vi "Position.vi"(0 "object in":refnum<class "5RobotsSkill.lvclass">, 2 "Robot":refnum<class "Robot.lvclass">, 4 "Game":refnum<class "Game.lvclass">, 5 "error in (no error)":errorcluster) -> (14 "object out":refnum<class "5RobotsSkill.lvclass">, 16 "Robot out":refnum<class "Robot.lvclass">, 19 "error out":errorcluster)   [LabVIEW 2024, in "5RobotsSkill.lvclass"]
uses:
  5RobotsSkill.lvclass
  Robot_class/Robot.lvclass
  Game_class/Game.lvclass
  Game_class/Game.lvclass/Game.ctl
  Robot_class/Robot.lvclass/Robot.ctl
  Robot_class/Read Zone.vi
  Robot_class/Write dest_orientation.vi
  Robot_class/Write dest_x.vi
  Robot_class/Write dest_y.vi
  Robot_class/Write kick_x.vi
  Robot_class/Write kick_z.vi
  Game_class/Read BallRef.vi
  Ball_class/Ball.lvclass
  Zone_class/Zone.lvclass
  Utilities_class/Utilities.lvclass
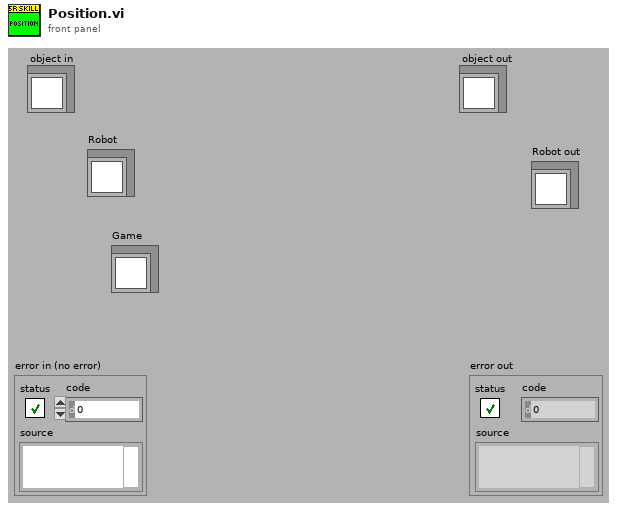
[diagram p1: front panel]
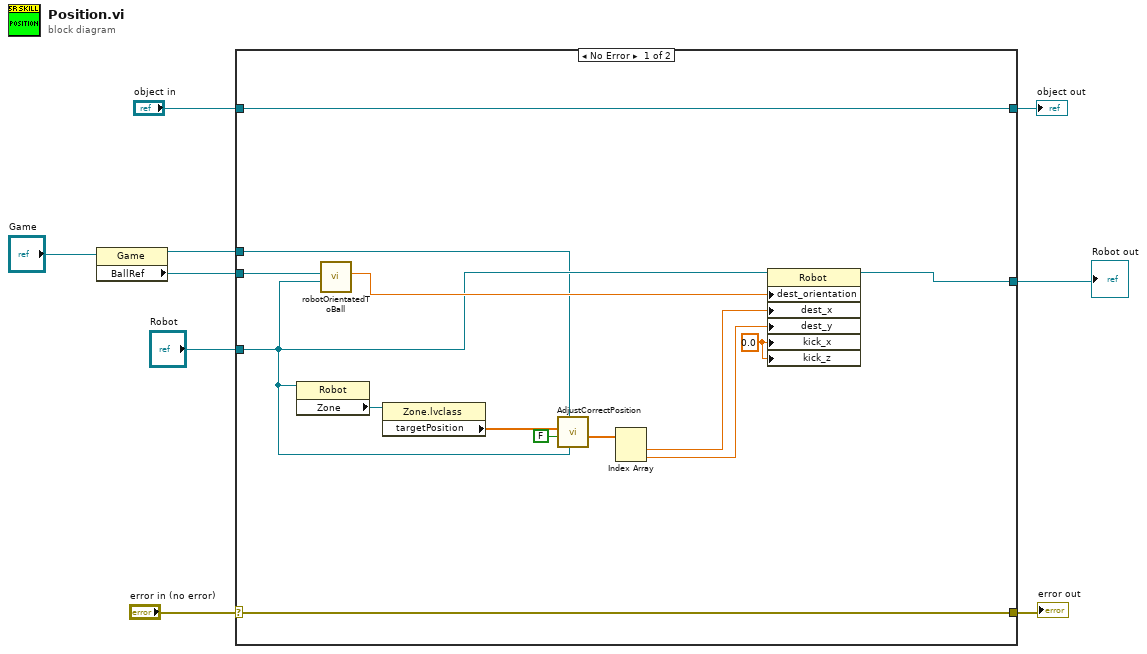
[diagram p0: block diagram]
diagram:
  n1 = property class="Game"(reference="Game") -> (reference out=w1:refnum<class "Game.lvclass">, "BallRef"=w2:refnum<class "Ball.lvclass">)  [unwired: 1 in, 1 out]
  n2 = case shown="No Error" "error in (no error)" {
    selector: "error in (no error)" -> [w22 w26]
    tunnel: [w22 w26] -> w8
    tunnel: [w23 w25] -> w6
    tunnel: "object in" -> [w23 w25]
    tunnel: "Robot" -> [w15 w24]
    tunnel: w2 -> [w21 _]
    tunnel: [w18 w24] -> w4
    tunnel: w1 -> [w11 _]
    frame No Error {
      w10 = 0.0 ("kick_x")
      n3 = property class="Robot"(reference=w15) -> ("Zone"=w19:refnum<class "Zone.lvclass">)  [unwired: 1 in, 2 out]
      n4 = call "robotOrientatedToBall.vi"("Robot"=w15, "BallRef"=w21) -> ("Orientation"=w20:dbl)  [unwired: 7 in, 2 out]
      n5 = property class="Zone.lvclass"(reference=w19) -> ("targetPosition"=w17:dbl[])  [unwired: 1 in, 2 out]
      n6 = call "AdjustCorrectPosition.vi"("Robot"=w15, "Game"=w11, "IsShoot?"=FALSE, "Position"=w17) -> ("AdjustPosition"=w14:dbl[])  [unwired: 5 in, 2 out]
      n7 = Index Array(array=w14) -> (element #1=w13:dbl, element #2=w12:dbl)  [unwired: 2 in]
      n8 = property class="Robot"(reference=w15, "dest_orientation"=w20, "dest_x"=w13, "dest_y"=w12, "kick_x"=w10, "kick_z"=w10) -> (reference out=w18:refnum<class "Robot.lvclass">)  [unwired: 1 in, 1 out]
    }
    frame Error {
    }
  }
  "error out" <- w8
  "object out" <- w6
  "Robot out" <- w4
